vi "Radar_Audio.vi"() -> ()   [LabVIEW 2014]
doc: "This VI illustrates how to acquire sound samples continuously from a specified device. It requires the use of a microphone attached to the sound card. You can specify the number of samples to acquire, sample rate, number of channels and a bit rate per sample. The VI also plots the raw data as the acquisition is made."
uses:
  <vilib>/sound2/lvsound2.llb/Sound Data Format.ctl
  <vilib>/sound2/lvsound2.llb/Sampling Mode.ctl
  <vilib>/sound2/lvsound2.llb/Sound Input Read (DBL).vi
panel:
  in  "start time":timestamp
  in  "stop time":timestamp
  in  "Save data":bool=TRUE caption="Enable"
  in  "Sound Format":T1={"sample rate (S/s)"=22050.0, "number of channels"=2, "bits per sample"=16}
  out "Raw Data":waveform(dbl)[](graph)
  in  "stop":bool
  in  "Device ID":u32 format="%.0x"
  in  "Number of Samples/ch":i32=5000
  # "Configuration"
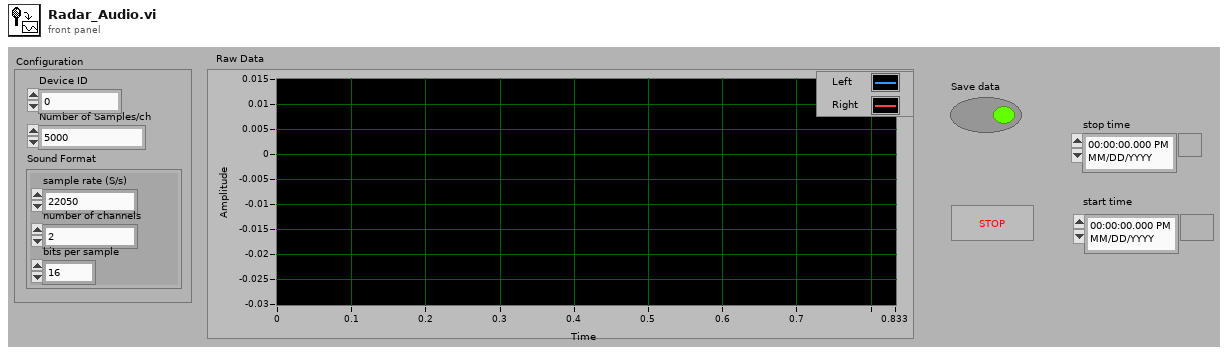
[diagram p1: front panel]
types:
  T1 = typedef "Sound Data Format.ctl" = cluster{"sample rate (S/s)":dbl, "number of channels":i32, "bits per sample":i32}
  T2 = typedef "Sampling Mode.ctl" = i32
  T3 = typedef "Sound Input Task ID.ctl" = u32
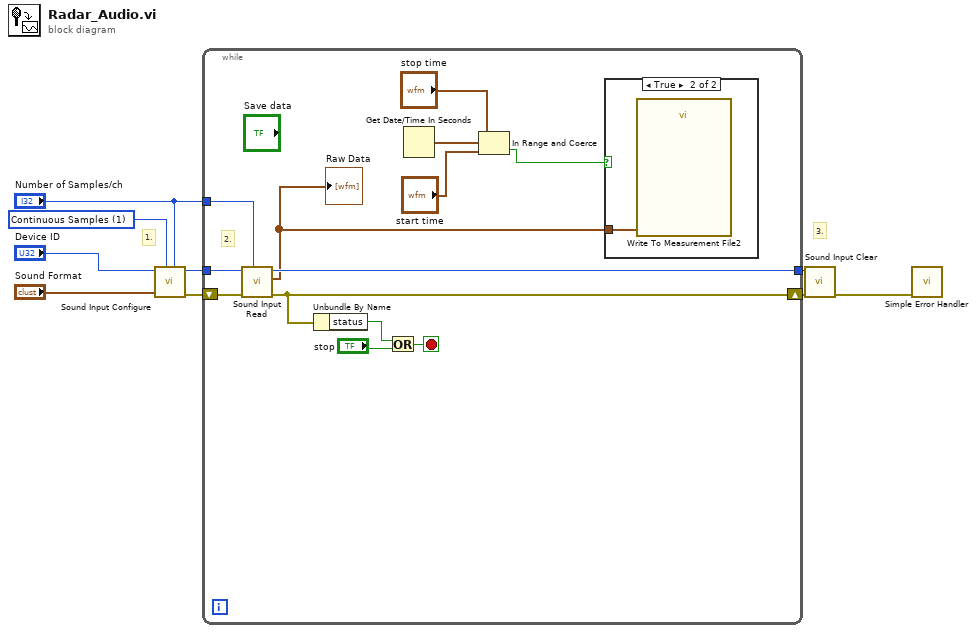
[diagram p0: block diagram]
diagram:
  w4 = T2 1 items=["Finite Samples", "Continuous Samples"] ("sample mode")
  # "3."
  # "1."
  n1 = call <vilib>:"Sound Input Configure.vi"("number of samples/ch"="Number of Samples/ch", "sample mode"=w4, "sound format"="Sound Format", "device ID"="Device ID") -> ("error out"=w9:errorcluster, "task ID"=w7:T3)  [unwired: 3 in, 3 out]
  n2 = while {
    tunnel: w7 -> [w21]
    tunnel: [w20] -> w6
    tunnel: "Number of Samples/ch" -> [w19]
    shift-right: [w15] -> w5
    shift-left: w9 -> [w22]
    stop <- w16 stop-if-true
    # "2."
    n3 = call-poly <vilib>:"Sound Input Read.vi"("number of samples/ch"=w19, "error in (no error)"=w22, "task ID"=w21) -> ("error out"=w15:errorcluster, "data"=w14:waveform(dbl)[], "task ID out"=w20:T3)  [unwired: 1 in, 5 out]
    "Raw Data" <- w14
    n4 = Unbundle By Name(w15) -> ("status"=w18:bool)
    n5 = Or(x=w18, y="stop") -> (x .or. y?=w16:bool)
    n6 = Get Date/Time In Seconds() -> (seconds since 1Jan1904=w13:timestamp)
    n7 = In Range and Coerce(upper limit="stop time", x=w13, lower limit="start time") -> (In Range?=w10:bool)  [unwired: 1 out]
    n8 = case shown="True" w10 {
      tunnel: w14 -> [_ w23]
      frame False {
      }
      frame True {
        n9 = call "Write To Measurement File2"("Signals"=w23) -> ()  [unwired: 16 in, 3 out]
      }
    }
  }
  n10 = call <vilib>:"Sound Input Clear.vi"("error in (no error)"=w5, "task ID"=w6) -> ("error out"=w2:errorcluster)  [unwired: 9 out]
  n11 = call <vilib>:"Simple Error Handler.vi"("error in (no error)"=w2) -> ()  [unwired: 1 in, 8 out]
